vi "Get Class Flags.vi"(8 "error in (no error)":errorcluster, 11 "Class ID":string="36") -> (0 "error out":errorcluster, 3 "Flags":cluster{"IsPrivate":bool, "IsScripting":bool})   [LabVIEW 2023]
doc: "<b> </b> <b> </b>\n© 2017 Q Software Innovations, LLC\nwritten by Quentin \"Q\" Alldredge\nproduced in LabVIEW 2015\n\nsupport@qsoftwareinnovations.com\nwww.qsoftwareinnovations.com\n\nAll rights reserved.\n\nRedistribution and use in source and binary forms, with or without modification, are permitted provided that the following conditions are met:\n\n * Redistributions of source code must retain the above copyright notice, this list of conditions and the following disclaimer.\n * Redistributions in binary form must reproduce the above copyright notice, this list of conditions and the following disclaimer in the documentation and/or other materials provided with the distribution.\n * Neither the name of Q Software Innovations, LLC. nor the names of its contributors may be used to endorse or promote products derived from this software without specific prior written permission.\n\nTHIS SOFTWARE IS PROVIDED BY THE COPYRIGHT HOLDERS AND CONTRIBUTORS \"AS IS\" AND ANY EXPRESS OR IMPLIED WARRANTIES, INCLUDING, BUT NOT LIMITED TO, THE IMPLIED WARRANTIES OF MERCHANTABILITY AND FITNESS FOR A PARTICULAR PURPOSE ARE DISCLAIMED. IN NO EVENT SHALL THE COPYRIGHT OWNER OR CONTRIBUTORS BE LIABLE FOR ANY DIRECT, INDIRECT, INCIDENTAL, SPECIAL, EXEMPLARY, OR CONSEQUENTIAL DAMAGES (INCLUDING, BUT NOT LIMITED TO, PROCUREMENT OF SUBSTITUTE GOODS OR SERVICES; LOSS OF USE, DATA, OR PROFITS; OR BUSINESS INTERRUPTION) HOWEVER CAUSED AND ON ANY THEORY OF LIABILITY, WHETHER IN CONTRACT, STRICT LIABILITY, OR TORT (INCLUDING NEGLIGENCE OR OTHERWISE) ARISING IN ANY WAY OUT OF THE USE OF THIS SOFTWARE, EVEN IF ADVISED OF THE POSSIBILITY OF SUCH DAMAGE."
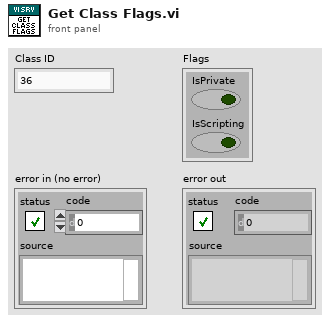
[diagram p1: front panel]
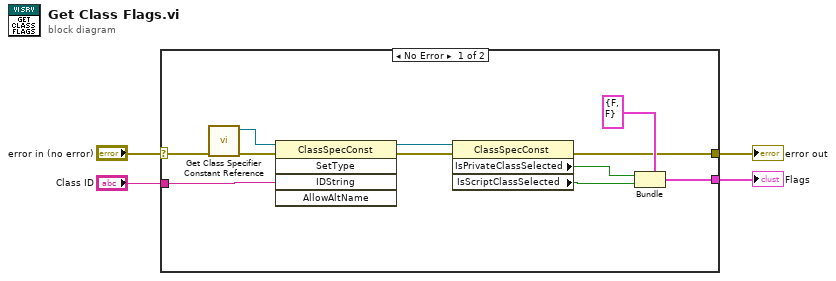
[diagram p0: block diagram]
diagram:
  n1 = case shown="No Error" "error in (no error)" {
    selector: "error in (no error)" -> [w15 w16]
    tunnel: [w7 w16] -> w3
    tunnel: "Class ID" -> [w12 _]
    tunnel: [w10 _] -> w1
    frame No Error {
      n2 = call "Get Class Specifier Constant Reference.vi"("error in (no error)"=w15) -> ("error out"=w13:errorcluster, "specific class reference"=w14:refnum<vi>)  [unwired: 9 in]
      n3 = invoke class="ClassSpecConst" method="SetType"(reference=w14, error in=w13, "IDString"=w12) -> (reference out=w9:refnum<vi>, error out=w11:errorcluster)  [unwired: 2 in, 3 out]
      n4 = property class="ClassSpecConst"(reference=w9, error in=w11) -> (error out=w7:errorcluster, "IsPrivateClassSelected"=w6:bool, "IsScriptClassSelected"=w5:bool)  [unwired: 1 out]
      n5 = Bundle(cluster=cluster{"IsPrivate":bool, "IsScripting":bool} {"IsPrivate"=FALSE, "IsScripting"=FALSE} ("Flags"), "IsPrivate"=w6, "IsScripting"=w5) -> (w10:cluster{"IsPrivate":bool, "IsScripting":bool})
    }
    frame Error {
    }
  }
  "error out" <- w3
  "Flags" <- w1
